vi "GetLogEntry.vi"(8 "error in":errorcluster, 11 "VISA Refnum in":refnum<visa-resource-name>) -> (0 "error out":errorcluster, 2 "Log Entry String":string, 3 "VISA Refnum out":refnum<visa-resource-name>)   [LabVIEW 2022 SP3]
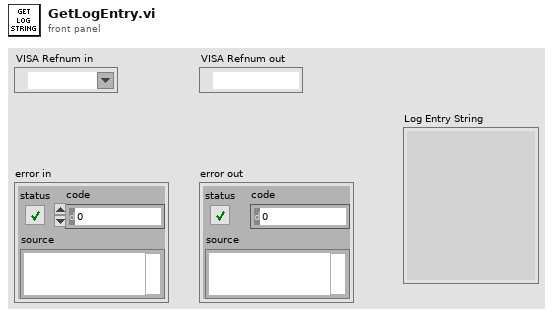
[diagram p1: front panel]
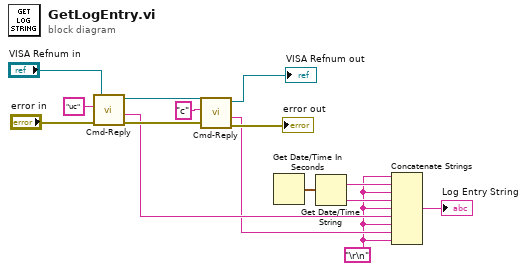
[diagram p0: block diagram]
diagram:
  w1 = "\r\n"
  n1 = call "Cmd-Reply.vi"("error in (no error)"="error in", "cmd"="uc" ("write buffer"), "VISA Refnum in"="VISA Refnum in") -> ("error out"=w13:errorcluster, "reply"=w8:string, "VISA Refnum out"=w12:refnum<visa-resource-name>)  [unwired: 6 in]
  n2 = call "Cmd-Reply.vi"("error in (no error)"=w13, "cmd"="c" ("write buffer"), "VISA Refnum in"=w12) -> ("error out"=→"error out":errorcluster, "reply"=w2:string, "VISA Refnum out"=→"VISA Refnum out":refnum<visa-resource-name>)  [unwired: 6 in]
  n3 = Get Date/Time In Seconds() -> (seconds since 1Jan1904=w4:timestamp)
  n4 = Get Date/Time String(seconds (now)=w4) -> (date string=w3:string, time string=w6:string)  [unwired: 2 in]
  n5 = Concatenate Strings(w1, w3, w1, w6, w1, w8, w1, w2, w1) -> (→"Log Entry String":string)
